vi "FindHostInfo.vi"(5 "responses":T3[](array[typedef]), 6 "error in":errorcluster) -> (0 "error out":errorcluster, 4 "hosts":T1[](array[typedef]))   [LabVIEW 2014, in "Autodetect.lvlib"]
uses:
  Autodetect.lvlib
  TypeDefs/UDP_Response_TD.ctl
  TypeDefs/UDP_HostinfoTD.ctl
  TypeDefs/HostTD.ctl
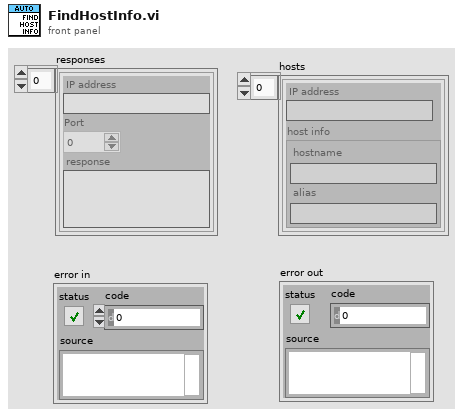
[diagram p1: front panel]
types:
  T1 = typedef "Autodetect.lvlib/HostTD.ctl" = cluster{"IP address":string, "host info":T2}
  T2 = typedef "Autodetect.lvlib/UDP_HostinfoTD.ctl" = cluster{"hostname":string, "alias":string}
  T3 = typedef "Autodetect.lvlib/UDP_Response_TD.ctl" = cluster{"IP address":string, "Port":u16, "response":string}
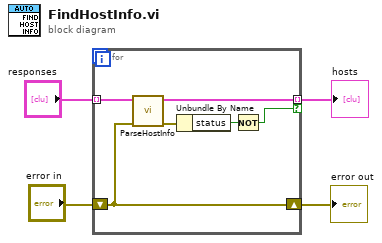
[diagram p0: block diagram]
diagram:
  n1 = for {
    tunnel: "responses" -> [w10] mode=indexing
    tunnel: [w9] -> w2 mode=indexing if=w7
    shift-right: [w5] -> w1
    shift-left: "error in" -> [w5]
    n2 = call "ParseHostInfo.vi"("error in (no error)"=w5, "response"=w10) -> ("error out"=w6:errorcluster, "Cluster"=w9:cluster{"IP address":string, "host info":T2})  [unwired: 8 in]
    n3 = Unbundle By Name(w6) -> ("status"=w8:bool)
    n4 = Not(x=w8) -> (.not. x?=w7:bool)
  }
  "hosts" <- w2
  "error out" <- w1
